vi "TdmsSaveData.vi"() -> ()   [LabVIEW 2010]
panel:
  out "App:Default Data Directory":path
  out "property value":i32
  out "Waveform Graph":waveform(dbl)[](graph)
  out "x-y":dbl
  out "data 2":dbl[](array[numeric])
  out "data":timestamp[](array[timestamp])
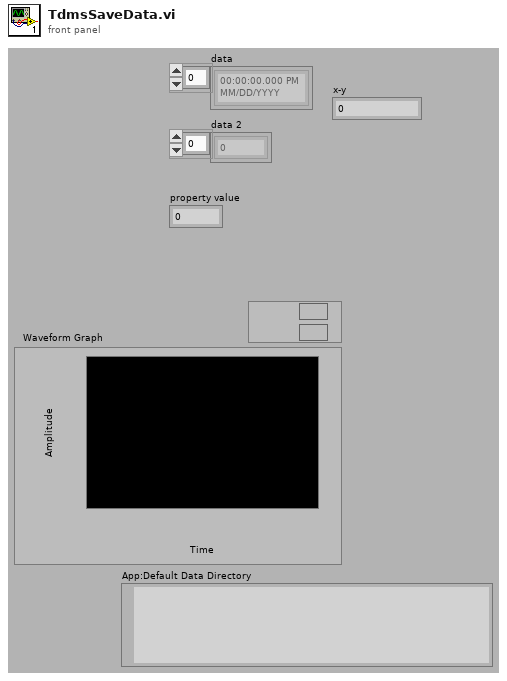
[diagram p1: front panel]
types:
  T1 = enum16{"open", "open or create", "create or replace", "create", "open (read-only)"}
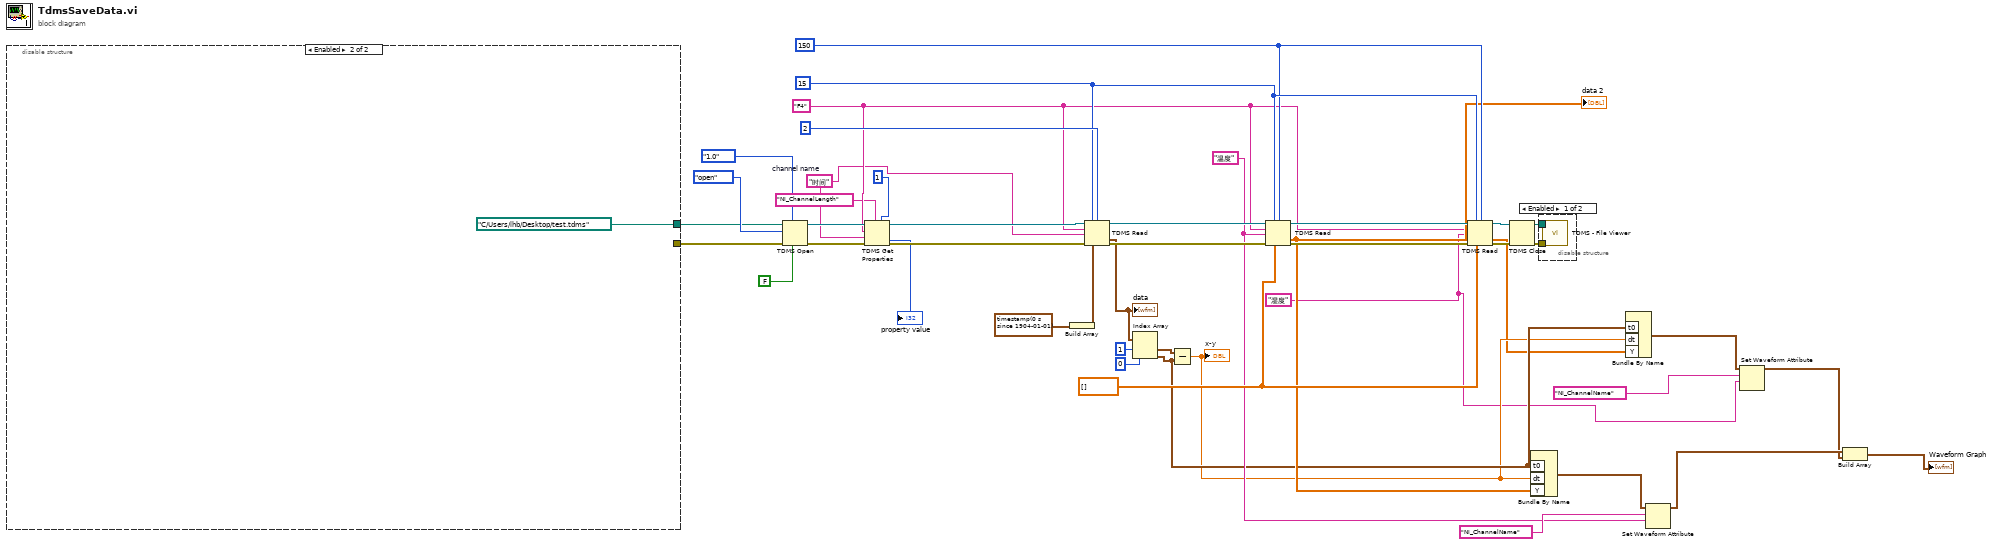
[diagram p0: block diagram]
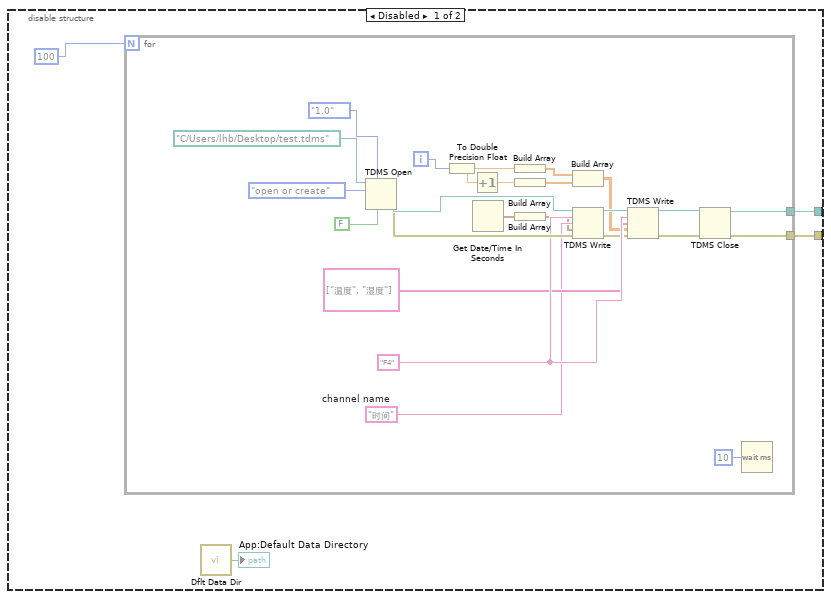
[diagram p2: hidden frame]
diagram:
  w1 = "时间"  # channel name
  w13 = "湿度"
  w27 = i64 150 ("count (-1: all)")
  w20 = "温度"
  w29 = dbl[] [] ("appended array")
  w28 = i64 15 ("offset (0)")
  w5 = "F4" ("group name in")
  n1 = disable-structure shown="Enabled" {
    disable-tunnel: [w49 path "C:/Users/lhb/Desktop/test.tdms" ("selected path")] -> w41
    disable-tunnel: [w48 _] -> w40
    frame Disabled {
      n2 = for {
        N: 100 -> [_]
        tunnel: [w62] -> w49
        tunnel: [w61] -> w48
        i -> [w50]
        w63 = "时间"  # channel name
        w66 = "F4" ("group name in (Untitled)")
        n3 = TDMS Open(6:FALSE ("disable buffering (T)"), 7:enum16{"1.0", "2.0"}."1.0" ("file format version (2.0)"), 10:T1."open or create" ("operation"), 11:path "C:/Users/lhb/Desktop/test.tdms" ("selected path")) -> (0:w69:errorcluster, 3:w70:refnum<k34>)  [unwired: 2 in]
        n4 = To Double Precision Float(number=w50) -> (double precision float=w52:dbl)
        n5 = Increment(x=w52) -> (x+1=w54:dbl)
        n6 = Get Date/Time In Seconds() -> (seconds since 1Jan1904=w60:timestamp)
        n7 = Build Array(w52) -> (w55:dbl[])
        n8 = Build Array(w54) -> (w53:dbl[])
        n9 = Build Array(w60) -> (w59:timestamp[])
        n10 = Build Array(w55, w53) -> (w56:dbl[][])
        n11 = TDMS Write(0:w70, 5:w66, 7:w63, 9:w59, 11:w69) -> (4:w58:refnum<k34>, 15:w57:errorcluster)  [unwired: 1 in, 2 out]
        n12 = TDMS Write(0:w58, 5:w66, 7:string[] ["温度", "湿度"] ("channel name(s) in (Untitled)"), 9:w56, 11:w57) -> (4:w73:refnum<k34>, 15:w72:errorcluster)  [unwired: 1 in, 2 out]
        n13 = TDMS Close(8:w72, 11:w73) -> (0:w61:errorcluster, 3:w62:path)
        n14 = Wait (ms)(milliseconds to wait=u32 10) -> ()  [unwired: 1 out]
      }
      n15 = call <vilib>:"Dflt Data Dir.vi"() -> ("App:Default Data Directory"=→"App:Default Data Directory":path)
    }
    frame Enabled {
    }
  }
  n16 = TDMS Open(6:FALSE ("disable buffering? (T)"), 7:enum16{"1.0", "2.0"}."1.0" ("file format version (2.0)"), 8:w40, 10:T1."open" ("operation (0:open)"), 11:w41) -> (0:w7:errorcluster, 3:w9:refnum<k34>)  [unwired: 1 in]
  n17 = TDMS Get Properties(5:1 ("index"), 7:"NI_ChannelLength" ("property name"), 8:w7, 9:w1, 10:w5, 11:w9) -> (0:w6:errorcluster, 3:w8:refnum<k34>, 4:→"property value":i32)  [unwired: 3 out]
  n18 = Build Array(timestamp(0 s since 1904-01-01) ("current time")) -> (w36:timestamp[])
  n19 = TDMS Read(0:w8, 1:w28, 2:i64 2 ("count (-1: all)"), 5:w5, 7:w1, 11:w6, 12:w36) -> (4:w32:refnum<k34>, 10:w23:timestamp[], 15:w35:errorcluster)  [unwired: 3 out]
  "data" <- w23
  n20 = Index Array(array=w23, index #1=1 ("index"), index #2=0 ("index")) -> (element #1=w24:timestamp, element #2=w16:timestamp)
  n21 = Subtract(x=w24, y=w16) -> (x-y=w15:dbl)
  "x-y" <- w15
  n22 = TDMS Read(0:w32, 1:w28, 2:w27, 5:w5, 7:w20, 11:w35, 12:w29) -> (4:w34:refnum<k34>, 10:w22:dbl[], 15:w33:errorcluster)  [unwired: 3 out]
  "data 2" <- w22
  n23 = TDMS Read(0:w34, 1:w28, 2:w27, 5:w5, 7:w13, 11:w33, 12:w29) -> (4:w31:refnum<k34>, 10:w14:dbl[], 15:w30:errorcluster)  [unwired: 3 out]
  n24 = TDMS Close(8:w30, 11:w31) -> (0:w38:errorcluster, 3:w39:path)
  n25 = Bundle By Name("t0"=w16, "dt"=w15, "Y"=w22) -> (w19:waveform(dbl))  [unwired: 1 in]
  n26 = disable-structure shown="Enabled" {
    disable-tunnel: w39 -> [w76 _]
    disable-tunnel: w38 -> [w75 _]
    frame Enabled {
      n27 = call <vilib>:"TDMS - File Viewer.vi"("error in (no error)"=w75, "file path"=w76) -> ()  [unwired: 6 out]
    }
    frame Disabled {
    }
  }
  n28 = Bundle By Name("t0"=w16, "dt"=w15, "Y"=w14) -> (w18:waveform(dbl))  [unwired: 1 in]
  n29 = Set Waveform Attribute(5:w20, 6:"NI_ChannelName" ("name"), 7:w19) -> (3:w12:waveform(dbl))  [unwired: 1 in, 2 out]
  n30 = Set Waveform Attribute(5:w13, 6:"NI_ChannelName" ("name"), 7:w18) -> (3:w11:waveform(dbl))  [unwired: 1 in, 2 out]
  n31 = Build Array(w12, w11) -> (→"Waveform Graph":waveform(dbl)[])
